vi "Generate Data.vi"(10 "Array in":i32[](array[numeric]), 11 "Array 3":dbl[](array[numeric])) -> (3 "Array out":dbl[][](array[numeric]))   [LabVIEW 2020]
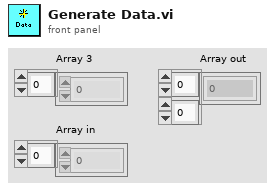
[diagram p1: front panel]
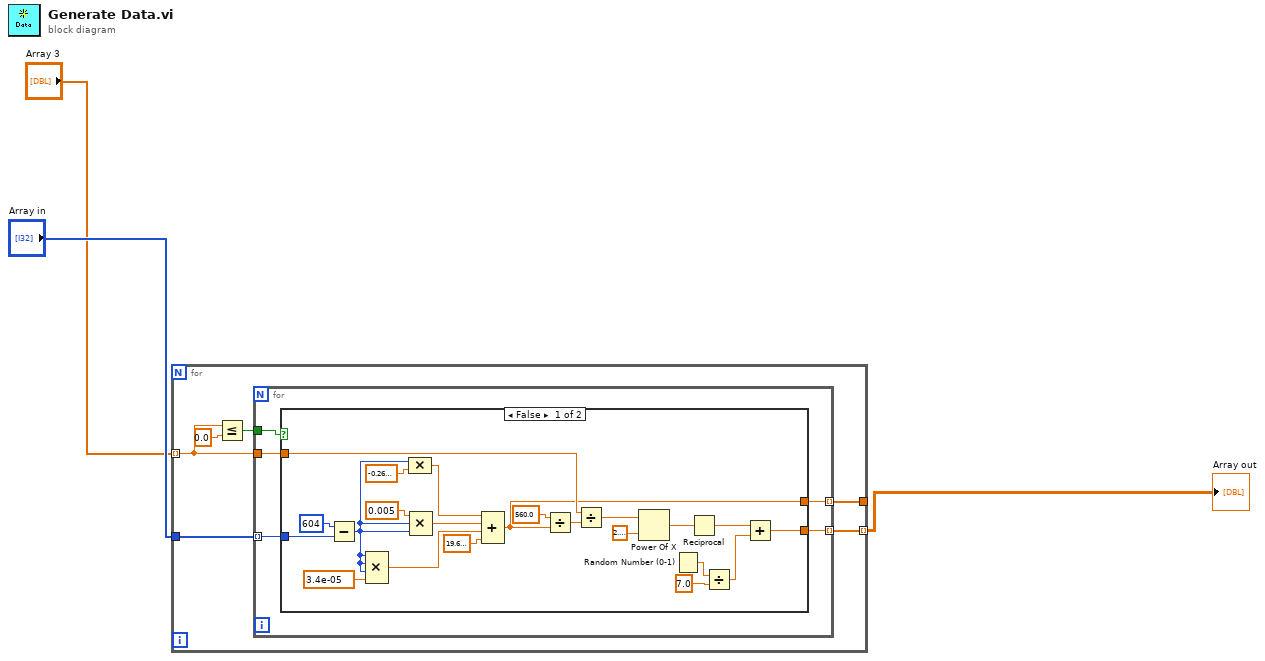
[diagram p0: block diagram]
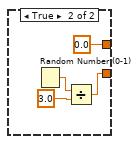
[diagram p2: hidden frame]
diagram:
  n1 = for {
    tunnel: "Array 3" -> [w6] mode=indexing
    tunnel: "Array in" -> [w8]
    tunnel: [w5] -> w2 mode=indexing
    tunnel: [w4] -> _
    n2 = Less Or Equal?(x=w6, y=0.0) -> (x <= y?=w7:bool)
    n3 = for {
      tunnel: w8 -> [w11] mode=indexing
      tunnel: w7 -> [w14]
      tunnel: w6 -> [w13]
      tunnel: [w12] -> w5 mode=indexing
      tunnel: [w10] -> w4 mode=indexing
      n4 = case shown="False" w14 {
        tunnel: w13 -> [w35 _]
        tunnel: [w19 w39] -> w12
        tunnel: w11 -> [w22 _]
        tunnel: [w23 0.0] -> w10
        frame False {
          n5 = Subtract(x=604 ("x 2"), y=w22) -> (x-y=w21:i32)
          n6 = Compound Arithmetic op=MULTIPLY(w21, w21, w21, 3.4e-05 ("a")) -> (w27:dbl)
          n7 = Compound Arithmetic op=MULTIPLY(w21, -0.26000000000000006 ("c")) -> (w29:dbl)
          n8 = Compound Arithmetic op=MULTIPLY(0.005 ("b"), w21, w21) -> (w28:dbl)
          n9 = Compound Arithmetic op=ADD(w29, w28, w27, 19.60000000000001 ("d")) -> (w23:dbl)
          n10 = Divide(x=560.0, y=w23) -> (x/y=w25:dbl)
          n11 = Divide(x=w35, y=w25) -> (x/y=w33:dbl)
          n12 = Power Of X(1:2.718281828459045, 2:w33) -> (0:w34:dbl)
          n13 = Random Number (0-1)() -> (number: 0 to 1=w17:dbl)
          n14 = Reciprocal(x=w34) -> (1/x=w18:dbl)
          n15 = Divide(x=w17, y=7.0) -> (x/y=w16:dbl)
          n16 = Add(x=w18, y=w16) -> (x+y=w19:dbl)
        }
        frame True {
          n17 = Random Number (0-1)() -> (number: 0 to 1=w40:dbl)
          n18 = Divide(x=w40, y=3.0) -> (x/y=w39:dbl)
        }
      }
    }
  }
  "Array out" <- w2
